vi "Get templates.vi"(8 "error in (no error)":errorcluster, 11 "Control in":refnum<class "Control.lvclass">) -> (0 "error out":errorcluster, 1 "CTL template":path, 2 "PNG templates":path[](array[path]), 3 "Control out":refnum<class "Control.lvclass">)   [LabVIEW 2012, in "Control.lvclass"]
doc: "Get the button templates from the template directory (LabVIEW Data folder)"
uses:
  Control.lvclass
  Control.lvclass/Control.ctl
  <userlib>/_OpenG.lib/string/string.llb/To Proper Case (String)__ogtk.vi
  <userlib>/_OpenG.lib/file/file.llb/Build Path - Traditional__ogtk.vi
  <userlib>/_OpenG.lib/file/file.llb/Build Path - File Names Array__ogtk.vi
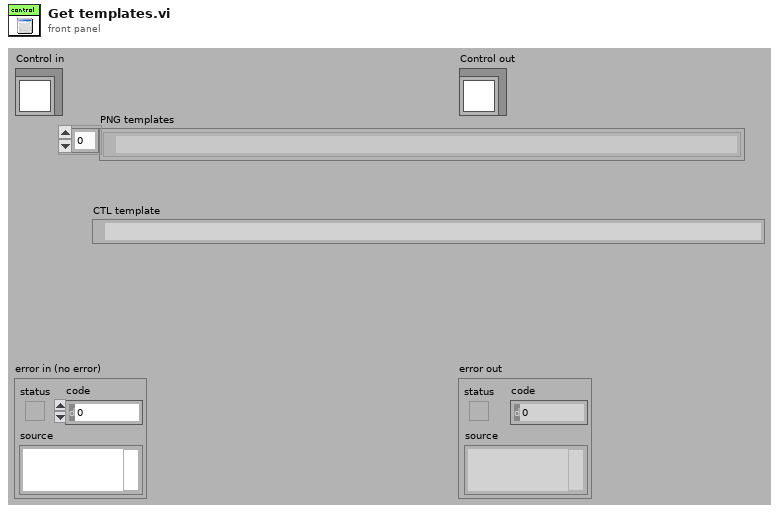
[diagram p1: front panel]
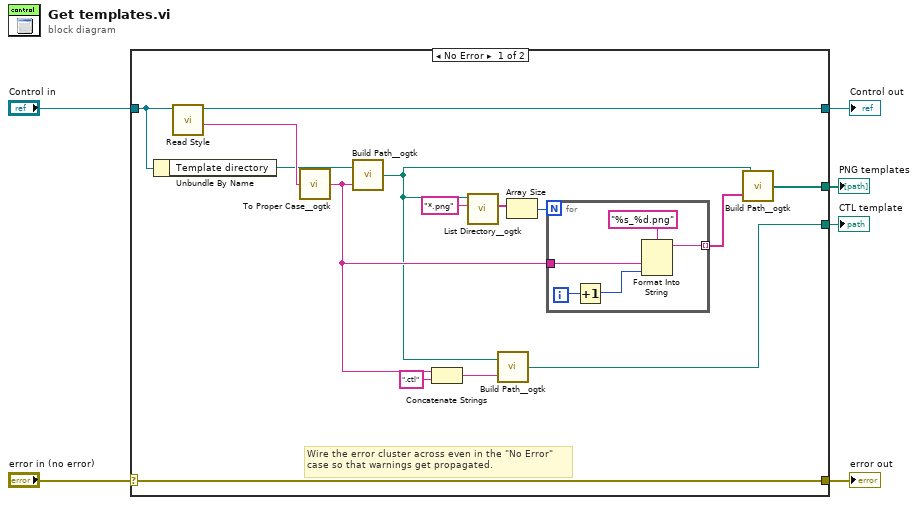
[diagram p0: block diagram]
diagram:
  n1 = case shown="No Error" "error in (no error)" {
    selector: "error in (no error)" -> [w21 w28]
    tunnel: [w21 w28] -> w5
    tunnel: [w13 w27] -> w3
    tunnel: "Control in" -> [w14 w27]
    tunnel: [w20 _] -> w2
    tunnel: [w15 _] -> w1
    frame No Error {
      # "Wire the error cluster across even in the \"No Error\"\ncase so that warnings get propagated."
      n2 = Unbundle By Name(w14) -> ("Template directory"=w11:path)
      n3 = call-dynamic "Read Style.vi"("Control in"=w14) -> ("Style name"=w12:string, "Control out"=w13:refnum<class "Control.lvclass">)  [unwired: 1 in, 8 out]
      n4 = call-poly <userlib>:"To Proper Case__ogtk.vi"("string"=w12) -> ("proper case string"=w17:string)  [unwired: 4 out]
      n5 = call-poly <userlib>:"Build Path__ogtk.vi"("name or relative path"=w17, "base path"=w11) -> ("appended path"=w7:path)
      n6 = Concatenate Strings(w17, ".ctl" ("string")) -> (w18:string)
      n7 = call <userlib>:"List Directory__ogtk.vi"("pattern"="*.png", "directory path"=w7) -> ("file names"=w9:string[])  [unwired: 1 in, 4 out]
      n8 = call-poly <userlib>:"Build Path__ogtk.vi"("name or relative path"=w18, "base path"=w7) -> ("appended path"=w15:path)
      n9 = Array Size(array=w9) -> (size(s)=w8:i32)
      n10 = for {
        N: w8 -> [_]
        tunnel: w17 -> [w24]
        tunnel: [w22] -> w16 mode=indexing
        i -> [w26]
        n11 = Increment(x=w26) -> (x+1=w25:i32)
        n12 = Format Into String(format string="%s_%d.png", w24, w25) -> (resulting string=w22:string)  [unwired: 2 in, 1 out]
      }
      n13 = call-poly <userlib>:"Build Path__ogtk.vi"("name or relative path"=w16, "base path"=w7) -> ("appended path"=w20:path[])
    }
    frame Error {
    }
  }
  "error out" <- w5
  "Control out" <- w3
  "PNG templates" <- w2
  "CTL template" <- w1
